vi "APC_PC_UI_Errors.vi"() -> ()   [LabVIEW 2020]
uses:
  controls/APC_ErrorCluster.ctl
  controls/APC_CylDaignosticsCluster.ctl
  <vilib>/Analysis/NI_AALBase.lvlib
panel:
  out "Clear warning request":bool
  in  "cycles for std":i32=100
  in  "Tab Control 2":enum32{"Main view", "Alternate view"}(tab)
  in  "Clear warnings":bool
  in  "Tab Control":T1(tab)=enum."CYLINDER"
  out "Round Color Box 5":u32[](array[colorbox])
  out "Round Color Box 4":u32[](array[colorbox])
  out "Round Color Box 3":u32[](array[colorbox])
  out "Round Color Box 2":u32[](array[colorbox])
  out "RASTER 5":string[](array[string])
  out "RASTER 4 : CRIO9056 : 9214-2 signals":string[](array[string])
  out "RASTER 3 : CRIO9056 : 9214-1 signals":string[](array[string])
  out "RASTER 2 : CRIO9056 : 9208 signals":string[](array[string])
  out "RASTER 1 : CRIO9056 : 9205 signals":string[](array[string])
  out "Round Color Box 1":u32[](array[colorbox])
  in  "ReloadINI9056":bool
  in  "MIN|MAX":i8[](array[numeric]) min=-1 max=1 step=1
  out "Measured value":dbl[](array[numeric])
  out "Selected raster":string[](array[string])
  in  "set9056":bool
  in  "retrieve9056":bool
  in  "Select raster":u8=1 min=1 max=5 step=1
  in  "ERROR level 2 : set IDLING":dbl[](array[numeric])
  out "Round Color Box selected":u32[](array[colorbox])
  in  "ERROR level 4: STOP and VENT":dbl[](array[numeric])
  in  "ERROR level 3 : set MOTORING":dbl[](array[numeric])
  in  "Soft WARNING level 1: self cleared":dbl[](array[numeric])
  in  "SaveINI9056":bool
  in  "Edit mode 9056":bool
  in  "Listbox":i32(listbox)
  in  "ReloadINI9049":bool
  out "s":dbl format="%#_4f"
  out "MAPO":dbl[](array[numeric])
  out "MAPO":dbl[][](graph)
  out "s":dbl format="%#_4f"
  out "s":dbl format="%#_4f"
  out "CA50":dbl[](array[numeric])
  out "CA50":dbl[][](graph)
  out "s":dbl format="%#_4f"
  out "Max p":dbl[][](graph)
  out "IMEP":dbl[][](graph)
  out "System error state":u32[][](array[colorbox])
  in  "Warning level : self cleared":dbl[](array[numeric])
  in  "Error level 2 : set MOTORING":dbl[](array[numeric])
  out "Selected raster 2":string[](array[string])=["Maximum pressure", "Misfire 1 (self reg)", "Misfire 2 (cyl to cyl)", "Misfire 3 (IMEPref)", "Cyclic variability", "MAPO", "Late combustion"]
  in  "Edit mode 9049":bool
  in  "SaveINI9049":bool
  in  "retrieve9049":bool
  in  "set9049":bool
  out "Waveform Graph":dbl[][](graph)
  out "IMEP":dbl[](array[numeric])
  out "IMEP s":dbl[](array[numeric]) format="%#.4f"
  out "Max p":dbl[](array[numeric])
  in  "EMERGENCY STOP":bool
  out "AI and system state":u32[][](array[colorbox])
  out "Cylinder pressure state":u32[][](array[colorbox])
  # "monarch APC v0.1"
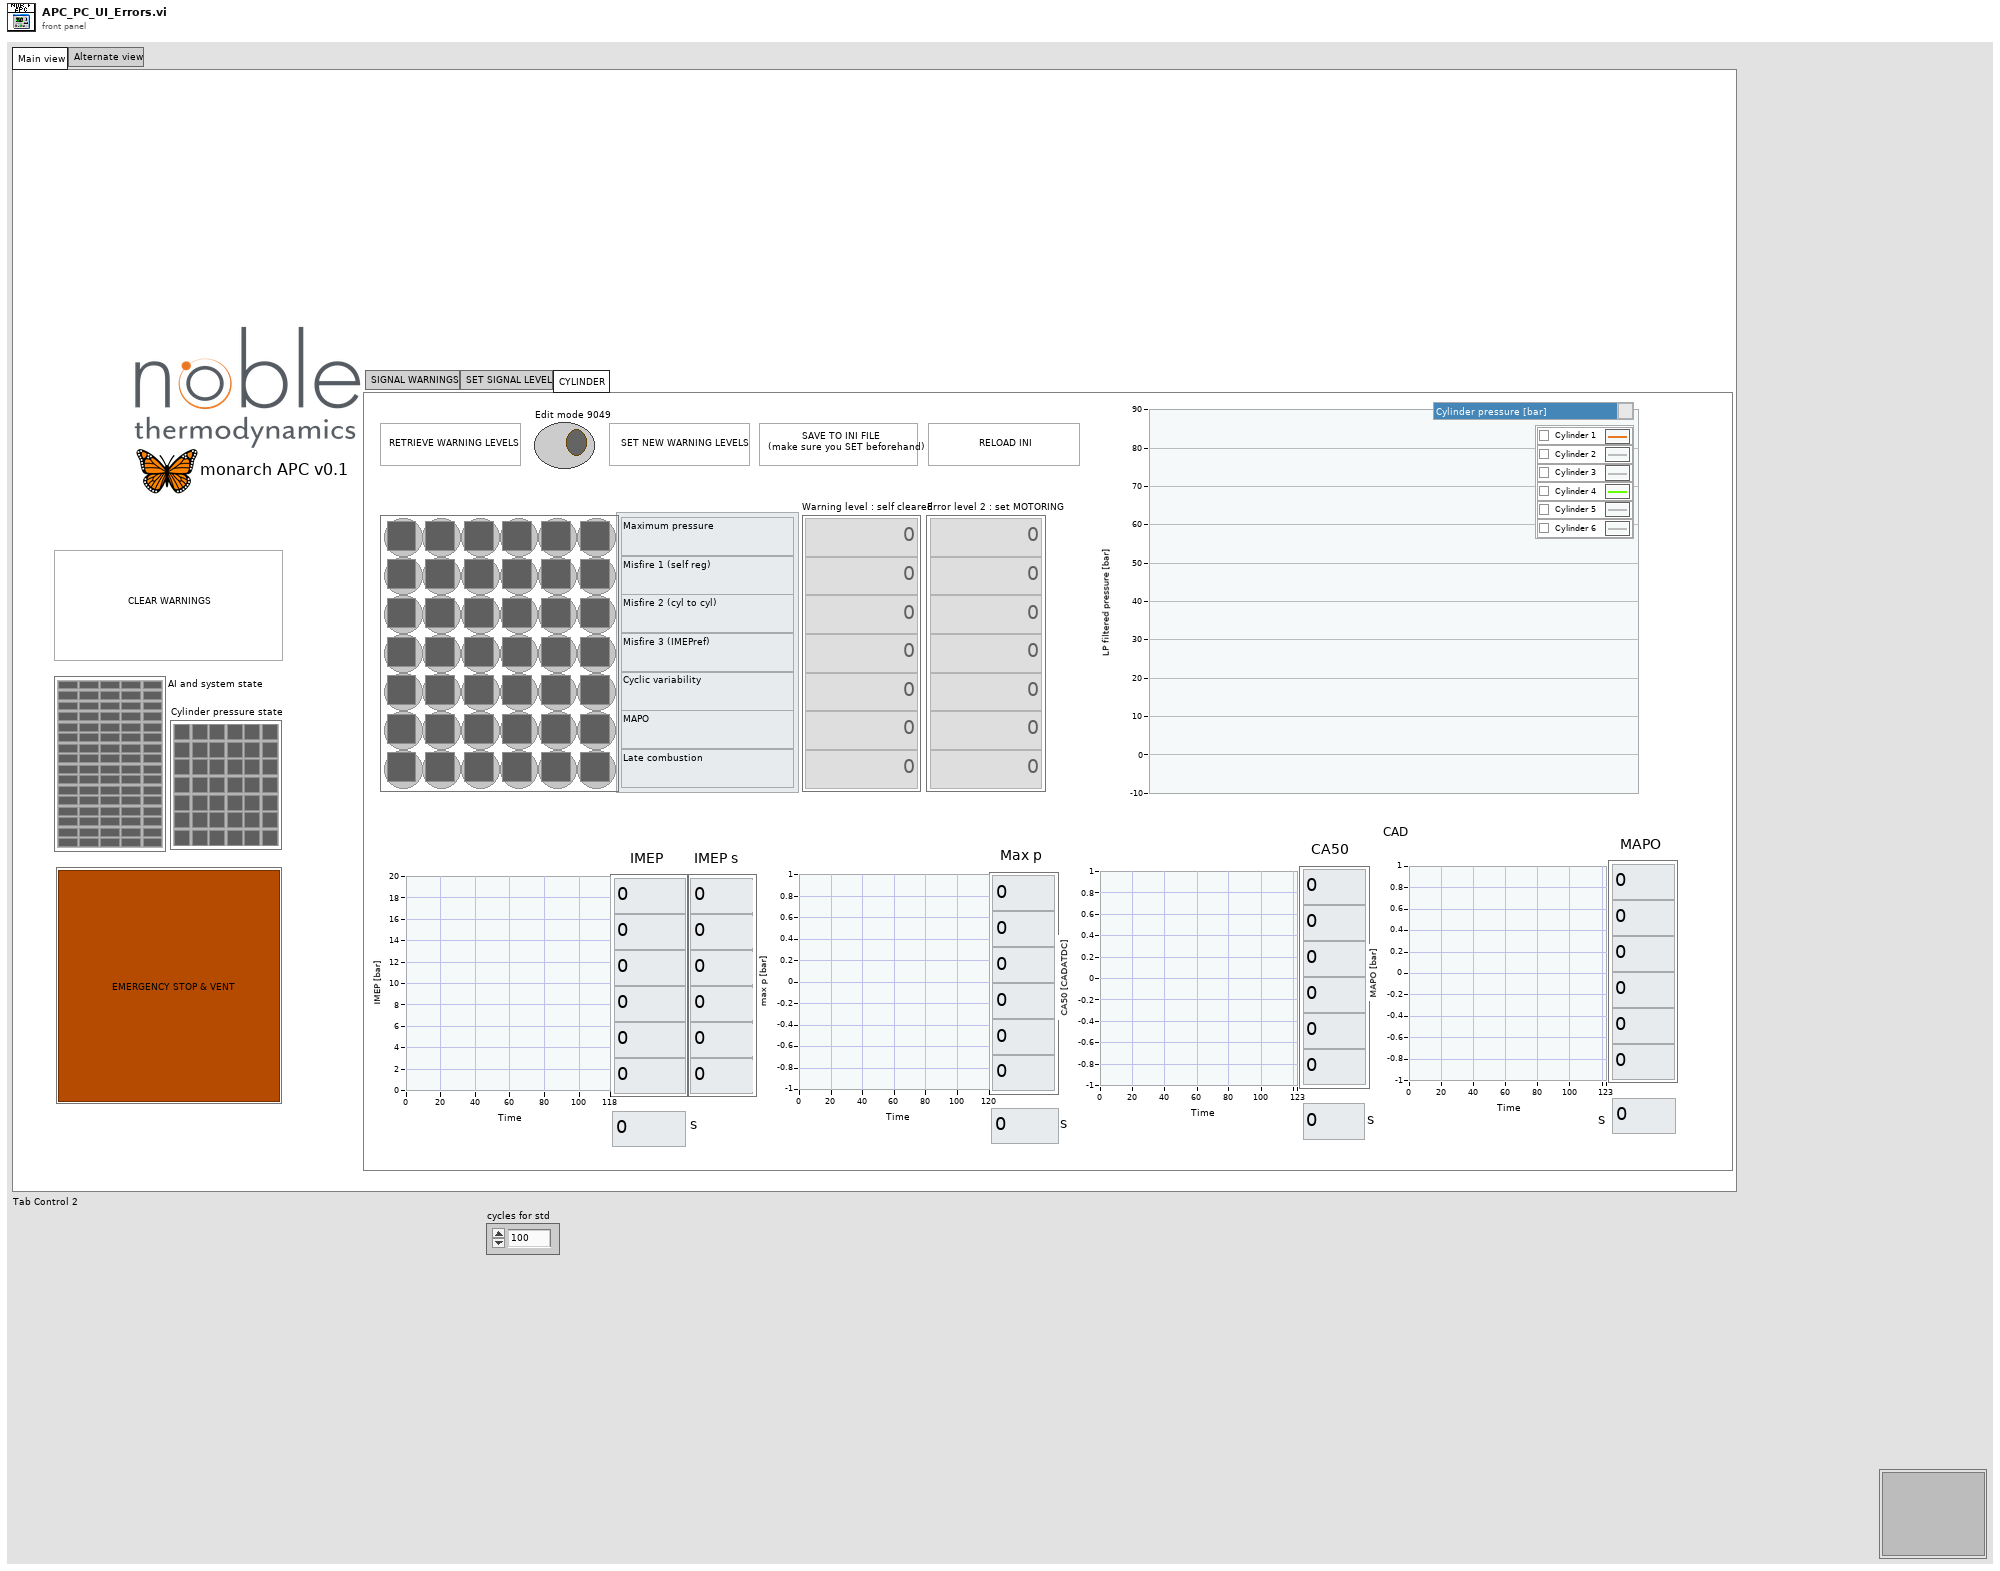
[diagram p1: front panel]
types:
  T1 = enum32{"SIGNAL WARNINGS", "SET SIGNAL LEVEL", "CYLINDER"}
  T2 = typedef "APC_ErrorCluster.ctl" = cluster{"AI and system state":u32[][], "Cylinder pressure state":u32[][], "EMERGENCY STOP":bool}
  T3 = typedef "APC_CylDaignosticsCluster.ctl" = cluster{"samples for running IMEP std":i32, "MaxDevFromExpectedIMEPError [bar]":dbl, "MaxDevFromExpectedIMEPWarning [bar]":dbl, "MaxDevFromAvgError [bar]":dbl, "MaxDevFromSelfAvgWarning [bar]":dbl, "MaxDevFromSelfAvgError [bar]":dbl, "MaxDevFromAvgWarning [bar]":dbl, "MaxIMEPstdWarning [bar]":dbl, "MaxIMEPstdError [bar]":dbl, "MAPOmaxError [bar/CAD]":dbl, "MAPOmaxWarning [bar/CAD]":dbl, "CA50maxError [CADATDC]":dbl, "CA50maxWarning [CADATDC]":dbl, "MaxPCylMaxError [bar]":dbl, "MaxPCylMaxWarning [bar]":dbl}
  T4 = typedef "APC_VisualizationCluster_v2.ctl" = cluster{"AR-FT-001":dbl, "AR-PT-001":dbl, "AR-TT-001":dbl, "AT103_CO2Conc":dbl, "AT201_CO2Conc":dbl, "C101_CompSpeed_rpm":dbl, "CO2 [%]":dbl, "EC-FC-001":dbl, "EC-TT-001":dbl, "EC-TT-002":dbl, "PC-TT-001":dbl, "PC-TT-002":dbl, "PC-TT-003":dbl, "PC-TT-004":dbl, "PC-TT-005":dbl, "PC-TT-006":dbl, "EO-PT-001":dbl, "EO-TT-001":dbl, "EO-TT-002":dbl, "FT301_Flow_kgh":dbl, "FV301_VlvPos_pc_fb":dbl, "IMEPn1":dbl, "IMEPn2":dbl, "IMEPn3":dbl, "IMEPn4":dbl, "IMEPn5":dbl, "IMEPn6":dbl, "IMEPstd1":dbl, "IMEPstd2":dbl, "IMEPstd3":dbl, "IMEPstd4":dbl, "IMEPstd5":dbl, "IMEPstd6":dbl, "NG-FC-001":dbl, "NG-FT-001":dbl, "NG-PT-001":dbl, "NG-TT-001":dbl, "NGDI-FT-001":dbl, "NGDI-PT-001":dbl, "NGDI-TT-001":dbl, "WF-OA-002-NOx":dbl, "TORQUE":dbl, "WF-OA-002-O2corr":dbl, "O2-FC-001":dbl, "O2-PT-001":dbl, "O2-TT-001":dbl, "PT103_Pressure_kPa":dbl, "PT104_Pressure_kPa":dbl, "PT106_Pressure_kPa":dbl, "PT300_Pressure_kPa":dbl, "PV103_VlvPos_pc_fb":dbl, "PV300_VlvPos_pc_fb":dbl, "MaxPcyl1":dbl, "MaxPcyl2":dbl, "MaxPcyl3":dbl, "MaxPcyl4":dbl, "MaxPcyl5":dbl, "MaxPcyl6":dbl, "SW-FC-004":dbl, "SW-FC-009":dbl, "SW-FT-001":dbl, "SW-FT-002":dbl, "SW-FT-003":dbl, "SW-FT-004":dbl, "SW-TT-001":dbl, "SW-TT-002":dbl, "SW-TT-003":dbl, "SW-TT-004":dbl, "SW-TT-005":dbl, "SW-TT-006":dbl, "SW-TT-007":dbl, "SW-TT-008":dbl, "WF-OA-001":dbl, "WF-OA-002":dbl, "WF-PT-001":dbl, "WF-PT-004":dbl, "WF-PT-005avg":dbl, "WF-PT-014":dbl, "WF-PT-015":dbl, "WF-PT-016":dbl, "WF-TT-001":dbl, "WF-TT-002":dbl, "WF-TT-003":dbl, "WF-TT-004":dbl, "WF-TT-007":dbl, "EngineSpeed_rpm":dbl, "SystemState":dbl, "CylPresWarnings":dbl, "CylPresErrors":dbl, "MAPO1":dbl, "MAPO2":dbl, "MAPO3":dbl, "MAPO4":dbl, "MAPO5":dbl, "MAPO6":dbl, "CA50_1":dbl, "CA50_2":dbl, "CA50_3":dbl, "CA50_4":dbl, "CA50_5":dbl, "CA50_6":dbl, "SparkTiming":dbl, "SW-TT-009":dbl, "NG-FV-001":dbl, "O2-PV-004":dbl, "AR-PV-004":dbl, "WF-FC-001":dbl, "WF-FC-002":dbl, "WF-FC-003":dbl, "WF-PT-012avg":dbl}
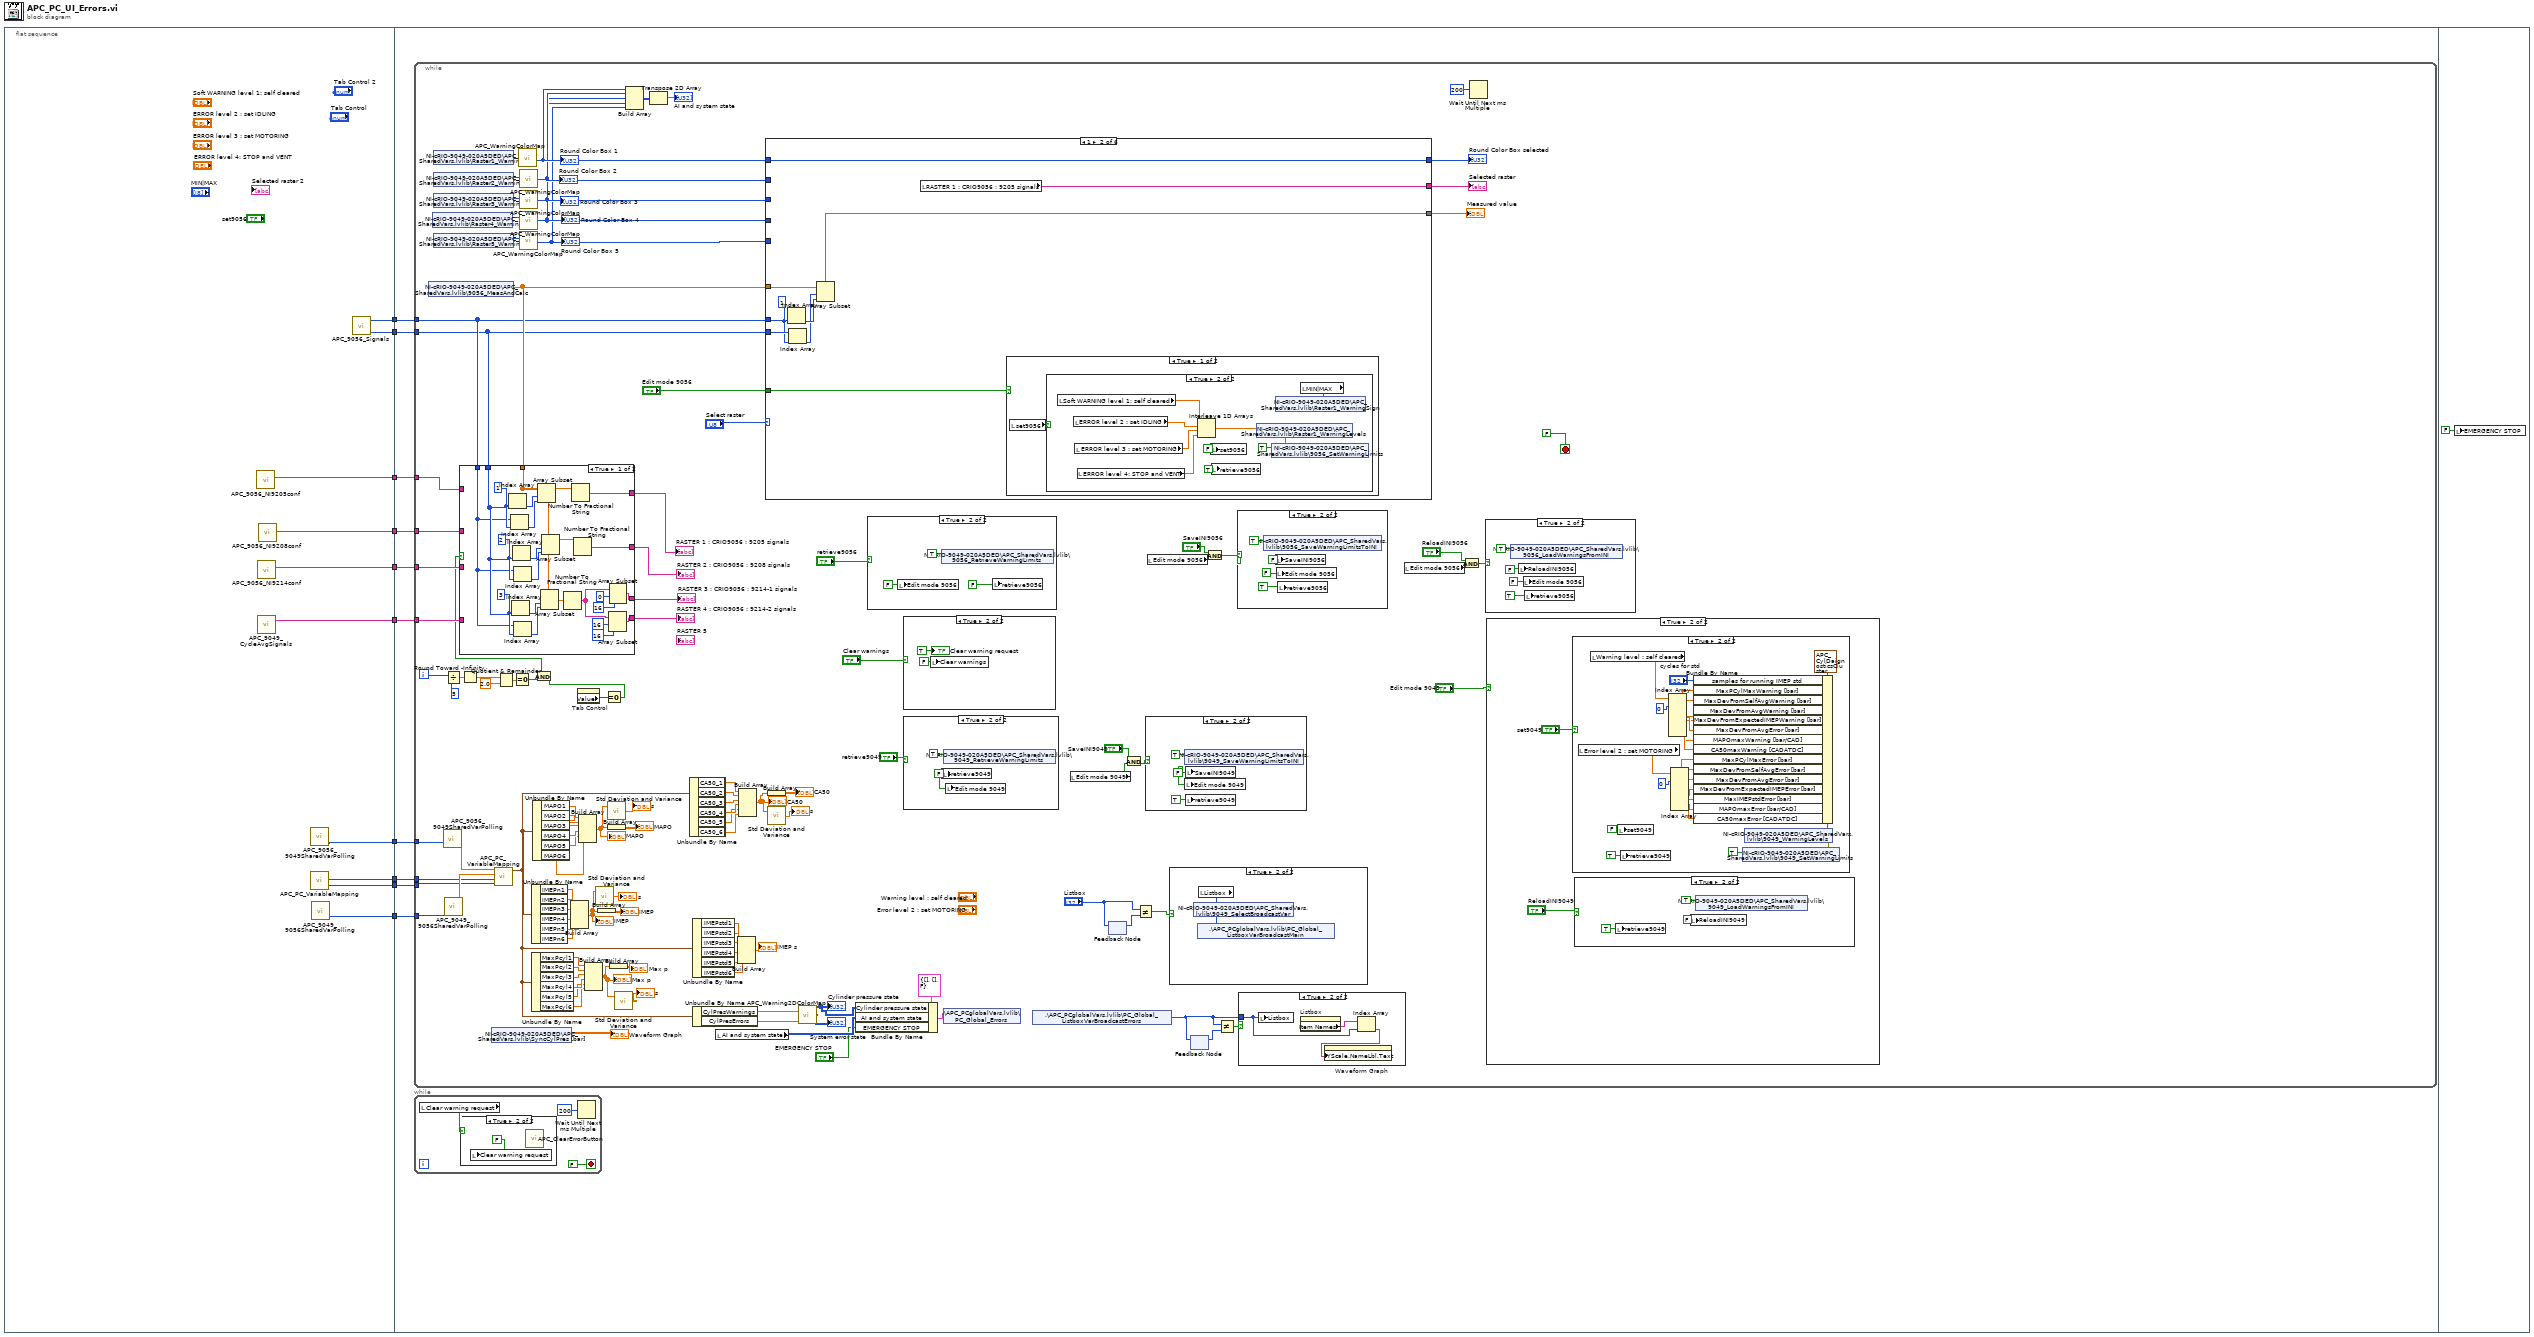
[diagram p0: block diagram]
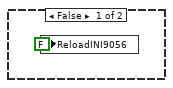
[diagram p5: hidden frame]
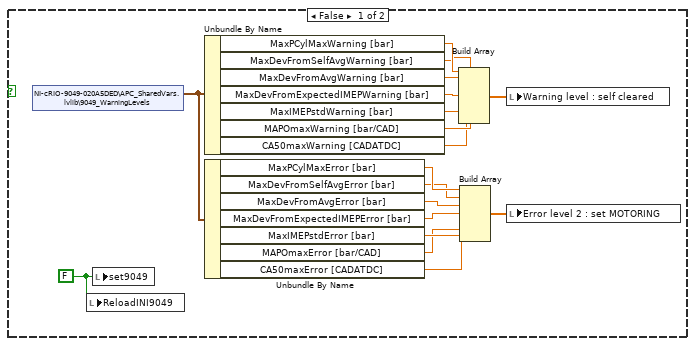
[diagram p6: hidden frame]
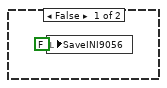
[diagram p13: hidden frame]
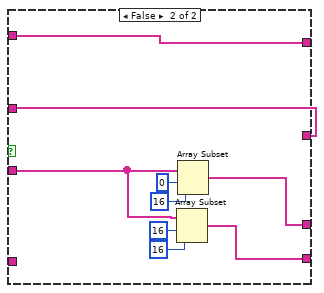
[diagram p14: hidden frame]
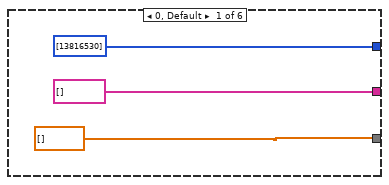
[diagram p15: hidden frame]
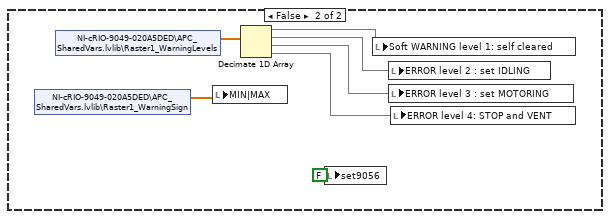
[diagram p17: hidden frame]
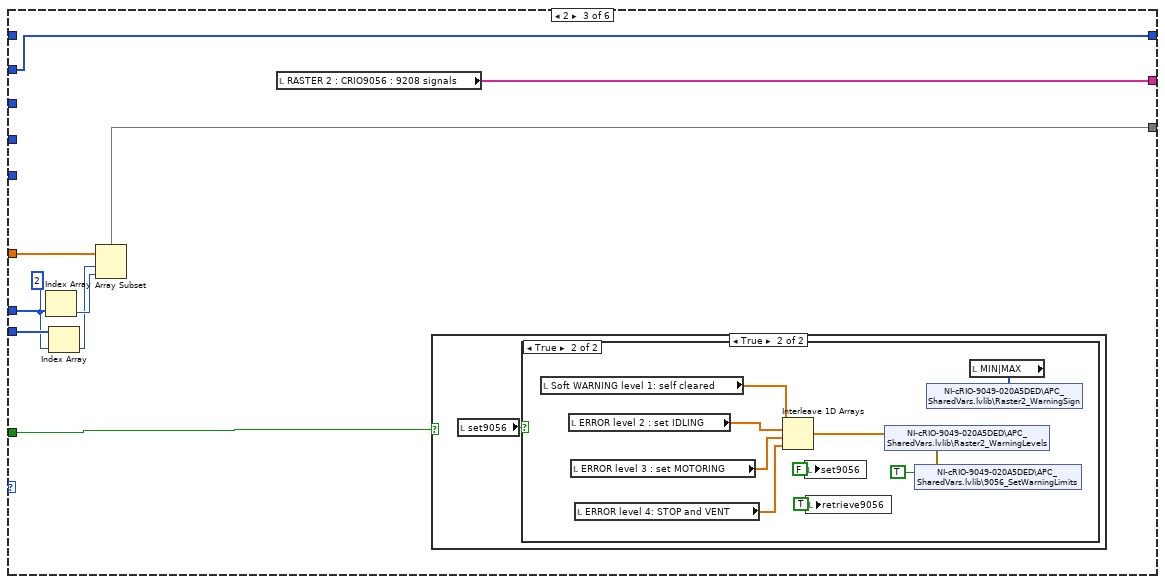
[diagram p18: hidden frame]
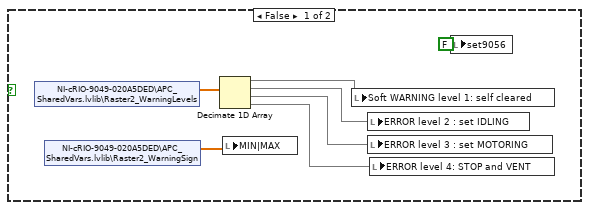
[diagram p19: hidden frame]
diagram:
  n1 = flat-sequence {
    tunnel: [w20] -> w10
    tunnel: [w19] -> w9
    tunnel: [w18] -> w8
    tunnel: [w17] -> w7
    tunnel: [w16] -> w6
    tunnel: [w15] -> w5
    tunnel: [w14] -> w4
    tunnel: [w13] -> w3
    tunnel: [w12] -> w2
    tunnel: [w11] -> w1
    tunnel: w10 -> [w30]
    tunnel: w9 -> [w29]
    tunnel: w8 -> [w28]
    tunnel: w7 -> [w27]
    tunnel: w6 -> [w26]
    tunnel: w5 -> [w25]
    tunnel: w4 -> [w24]
    tunnel: w3 -> [w23]
    tunnel: w2 -> [w22]
    tunnel: w1 -> [w21]
    frame #0 {
      n2 = call "APC_9056_NI9205conf.vi"() -> ("channels name out"=w18:string[])  [unwired: 5 out]
      n3 = call "APC_9056_NI9214conf.vi"() -> ("channels name out"=w16:string[])  [unwired: 5 in]
      n4 = call "APC_9049_CycleAvgSignals.vi"() -> ("CRIo9049_CycleAvgSignals"=w15:string[])  [unwired: 3 in]
      n5 = call "APC_9056_NI9208conf.vi"() -> ("channels name out"=w17:string[])  [unwired: 5 out]
      n6 = call "APC_9056_9049SharedVarPolling.vi"() -> ("Number of signals (out)"=w14:i32)  [unwired: 1 in, 1 out]
      n7 = call "APC_PC_VariableMapping.vi"() -> ("Index 9056"=w11:i32[], "Index 9049"=w12:i32[])  [unwired: 4 in, 1 out]
      n8 = call "APC_9049_9056SharedVarPolling.vi"() -> ("Number of signals (out)"=w13:i32)  [unwired: 1 in, 3 out]
      n9 = call "APC_9056_Signals.vi"() -> ("Starting Index"=w19:i32[], "signals per group"=w20:i32[])  [unwired: 3 in, 1 out]
    }
    frame #1 {
      n10 = while {
        tunnel: w30 -> [w124]
        tunnel: w29 -> [w123]
        tunnel: w28 -> [w136]
        tunnel: w27 -> [w135]
        tunnel: w26 -> [w134]
        tunnel: w25 -> [w133]
        tunnel: w24 -> [w114]
        tunnel: w23 -> [w113]
        tunnel: w22 -> [w112]
        tunnel: w21 -> [w111]
        i -> [w142]
        stop <- FALSE stop-if-true
        n11 = shared-variable "NI-cRIO-9049-020A5DED\\APC_SharedVars.lvlib\\9056_MeasAndCalc"() -> (w128:dbl[])  [unwired: 1 in, 1 out]
        n12 = shared-variable "NI-cRIO-9049-020A5DED\\APC_SharedVars.lvlib\\Raster4_Warnings"() -> (w146:u8[])  [unwired: 1 in, 1 out]
        n13 = shared-variable "NI-cRIO-9049-020A5DED\\APC_SharedVars.lvlib\\Raster1_Warnings"() -> (w149:u8[])  [unwired: 1 in, 1 out]
        n14 = shared-variable "NI-cRIO-9049-020A5DED\\APC_SharedVars.lvlib\\Raster2_Warnings"() -> (w148:u8[])  [unwired: 1 in, 1 out]
        n15 = shared-variable "NI-cRIO-9049-020A5DED\\APC_SharedVars.lvlib\\Raster3_Warnings"() -> (w147:u8[])  [unwired: 1 in, 1 out]
        n16 = shared-variable "NI-cRIO-9049-020A5DED\\APC_SharedVars.lvlib\\Raster5_Warnings"() -> (w145:u8[])  [unwired: 1 in, 1 out]
        n17 = call "APC_9056_9049SharedVarPolling.vi"("Number of signals"=w114) -> ("9049_CycleAveragedVariables"=w116:dbl[])  [unwired: 1 out]
        n18 = call "APC_9049_9056SharedVarPolling.vi"("Number of signals"=w113) -> ("9056 IO"=w115:dbl[])  [unwired: 3 out]
        n19 = Divide(x=w142, y=5) -> (x/y=w140:dbl)
        n20 = Round Toward -Infinity(1:w140) -> (0:w139:dbl)
        n21 = shared-variable "NI-cRIO-9049-020A5DED\\APC_SharedVars.lvlib\\SyncCylPres [bar]"() -> (→"Waveform Graph":dbl[][])  [unwired: 1 in, 1 out]
        n22 = call "APC_PC_VariableMapping.vi"("Index of array for 9056"=w111, "Index of array for 9049"=w112, "9056 IO"=w115, "9049_CycleAveragedVariables"=w116) -> ("Output cluster"=w85:T4)  [unwired: 2 out]
        n23 = Quotient & Remainder(x=w139, y=2.0) -> (x-y*floor(x/y)=w137:dbl)  [unwired: 1 out]
        n24 = Equal To 0?(x=w137) -> (x = 0?=w127:bool)
        n25 = call "APC_WarningColorMap.vi"("Array"=w149) -> ("Round Color Box"=w67:u32[])
        "Round Color Box 1" <- w67
        n26 = call "APC_WarningColorMap.vi"("Array"=w148) -> ("Round Color Box"=w66:u32[])
        "Round Color Box 2" <- w66
        n27 = call "APC_WarningColorMap.vi"("Array"=w147) -> ("Round Color Box"=w65:u32[])
        "Round Color Box 3" <- w65
        n28 = call "APC_WarningColorMap.vi"("Array"=w146) -> ("Round Color Box"=w64:u32[])
        "Round Color Box 4" <- w64
        n29 = call "APC_WarningColorMap.vi"("Array"=w145) -> ("Round Color Box"=w63:u32[])
        "Round Color Box 5" <- w63
        n30 = Unbundle By Name(w85) -> ("IMEPn1"=w109:dbl, "IMEPn2"=w104:dbl, "IMEPn3"=w105:dbl, "IMEPn4"=w106:dbl, "IMEPn5"=w107:dbl, "IMEPn6"=w108:dbl)
        n31 = Unbundle By Name(w85) -> ("MaxPcyl1"=w96:dbl, "MaxPcyl2"=w95:dbl, "MaxPcyl3"=w94:dbl, "MaxPcyl4"=w93:dbl, "MaxPcyl5"=w92:dbl, "MaxPcyl6"=w91:dbl)
        n32 = Unbundle By Name(w85) -> ("MAPO1"=w83:dbl, "MAPO2"=w82:dbl, "MAPO3"=w81:dbl, "MAPO4"=w80:dbl, "MAPO5"=w79:dbl, "MAPO6"=w78:dbl)
        n33 = Build Array(w109, w104, w105, w106, w107, w108) -> (w60:dbl[])
        "IMEP" <- w60
        n34 = property on="Tab Control" class="TabCtl (strict)"() -> ("Value"=w121:T1)  [unwired: 2 in, 2 out]
        n35 = Build Array(w83, w82, w81, w80, w79, w78) -> (w47:dbl[])
        "MAPO" <- w47
        n36 = Build Array(w96, w95, w94, w93, w92, w91) -> (w43:dbl[])
        "Max p" <- w43
        n37 = call <vilib>:"Std Deviation and Variance.vi"("X"=w60) -> ("standard deviation"=→"s":dbl)  [unwired: 1 in, 2 out]
        n38 = Build Array(w60) -> (→"IMEP":dbl[][])
        n39 = Equal To 0?(x=w121) -> (x = 0?=w125:bool)
        n40 = And(x=w125, y=w127) -> (x .and. y?=w126:bool)
        n41 = case shown="True" w126 {
          tunnel: [w234 w256] -> w132
          tunnel: w136 -> [_ w256]
          tunnel: [w232 w255] -> w131
          tunnel: w135 -> [_ w255]
          tunnel: [w224 w254] -> w130
          tunnel: w134 -> [_ w249]
          tunnel: [w225 w248] -> w129
          tunnel: w133 -> [_ _]
          tunnel: w128 -> [w236 _]
          tunnel: w123 -> [w238 _]
          tunnel: w124 -> [w237 _]
          frame True {
            w239 = 3 ("index")
            w242 = 2 ("index")
            w245 = 1 ("index")
            n42 = Index Array(array=w238, index=w245) -> (element=w247:i32)
            n43 = Index Array(array=w237, index=w245) -> (element=w246:i32)
            n44 = Index Array(array=w238, index=w239) -> (element=w241:i32)
            n45 = Index Array(array=w238, index=w242) -> (element=w244:i32)
            n46 = Index Array(array=w237, index=w239) -> (element=w240:i32)
            n47 = Index Array(array=w237, index=w242) -> (element=w243:i32)
            n48 = Array Subset(array=w236, index=w247, length=w246) -> (w235:dbl[])
            n49 = Array Subset(array=w236, index=w241, length=w240) -> (w231:dbl[])
            n50 = Array Subset(array=w236, index=w244, length=w243) -> (w233:dbl[])
            n51 = Number To Fractional String(number=w231) -> (F-format string=w226:string[])  [unwired: 3 in]
            n52 = Number To Fractional String(number=w235) -> (F-format string=w234:string[])  [unwired: 3 in]
            n53 = Number To Fractional String(number=w233) -> (F-format string=w232:string[])  [unwired: 3 in]
            n54 = Array Subset(array=w226, index=16, length=16) -> (w225:string[])
            n55 = Array Subset(array=w226, index=0, length=16) -> (w224:string[])
          }
          frame False {
            n56 = Array Subset(array=w249, index=16, length=16) -> (w248:string[])
            n57 = Array Subset(array=w249, index=0, length=16) -> (w254:string[])
          }
        }
        "RASTER 1 : CRIO9056 : 9205 signals" <- w132
        "RASTER 2 : CRIO9056 : 9208 signals" <- w131
        "RASTER 3 : CRIO9056 : 9214-1 signals" <- w130
        "RASTER 4 : CRIO9056 : 9214-2 signals" <- w129
        n58 = Build Array(w47) -> (→"MAPO":dbl[][])
        n59 = call <vilib>:"Std Deviation and Variance.vi"("X"=w47) -> ("standard deviation"=→"s":dbl)  [unwired: 1 in, 2 out]
        n60 = Build Array(w43) -> (→"Max p":dbl[][])
        n61 = call <vilib>:"Std Deviation and Variance.vi"("X"=w43) -> ("standard deviation"=→"s":dbl)  [unwired: 1 in, 2 out]
        n62 = Build Array(w67, w66, w65, w64, w63) -> (w62:u32[][])
        n63 = Transpose 2D Array(2D array=w62) -> (transposed array=→"AI and system state":u32[][])
        n64 = Unbundle By Name(w85) -> ("CA50_1"=w84:dbl, "CA50_2"=w90:dbl, "CA50_3"=w89:dbl, "CA50_4"=w88:dbl, "CA50_5"=w87:dbl, "CA50_6"=w86:dbl)
        n65 = Unbundle By Name(w85) -> ("IMEPstd1"=w103:dbl, "IMEPstd2"=w102:dbl, "IMEPstd3"=w101:dbl, "IMEPstd4"=w100:dbl, "IMEPstd5"=w99:dbl, "IMEPstd6"=w98:dbl)
        n66 = Unbundle By Name(w85) -> ("CylPresWarnings"=w77:dbl, "CylPresErrors"=w76:dbl)
        n67 = local read "AI and system state"() -> (w39:u32[][])
        n68 = Build Array(w103, w102, w101, w100, w99, w98) -> (→"IMEP s":dbl[])
        n69 = Build Array(w84, w90, w89, w88, w87, w86) -> (w46:dbl[])
        "CA50" <- w46
        n70 = case shown="1" "Select raster" {
          tunnel: w67 -> [_ w269 _ _ _ _]
          tunnel: w66 -> [_ _ w289 _ _ _]
          tunnel: w65 -> [_ _ _ w318 _ _]
          tunnel: w64 -> [_ _ _ _ w349 _]
          tunnel: w63 -> [_ _ _ _ _ w375]
          tunnel: [u32[] [13816530] ("Round Color Box") w269 w289 w318 w349 w375] -> w150
          tunnel: [string[] [] ("RASTER 5") w268 w297 w325 w355 w383] -> w144
          tunnel: [dbl[] [] ("Measured value") w263 w292 w320 w350 w378] -> w143
          tunnel: w128 -> [_ w267 w296 w324 w354 w382]
          tunnel: w124 -> [_ w266 w295 w323 w353 w381]
          tunnel: w123 -> [_ w265 w294 w322 w352 w380]
          tunnel: "Edit mode 9056" -> [_ w260 w288 w317 w348 w374]
          frame 0, Default {
          }
          frame 1 {
            w264 = 1 ("index")
            n71 = Index Array(array=w266, index=w264) -> (element=w262:i32)
            n72 = Index Array(array=w265, index=w264) -> (element=w261:i32)
            n73 = Array Subset(array=w267, index=w261, length=w262) -> (w263:dbl[])
            n74 = local read "RASTER 1 : CRIO9056 : 9205 signals"() -> (w268:string[])
            n75 = case shown="True" w260 {
              frame True {
                n76 = local read "set9056"() -> (w270:bool)
                n77 = case shown="True" w270 {
                  frame False {
                  }
                  frame True {
                    n78 = local read "Soft WARNING level 1: self cleared"() -> (w276:dbl[])
                    n79 = local read "ERROR level 2 : set IDLING"() -> (w275:dbl[])
                    n80 = local read "ERROR level 3 : set MOTORING"() -> (w274:dbl[])
                    n81 = local read "ERROR level 4: STOP and VENT"() -> (w273:dbl[])
                    n82 = Interleave 1D Arrays(w276, w275, w274, w273) -> (w272:dbl[])
                    n83 = local write "set9056"(FALSE ("set")) -> ()
                    n84 = local write "retrieve9056"(TRUE ("retrieve")) -> ()
                    n85 = shared-variable "NI-cRIO-9049-020A5DED\\APC_SharedVars.lvlib\\Raster1_WarningLevels"(w272) -> (error out=w277:errorcluster)  [unwired: 1 in]
                    n86 = shared-variable "NI-cRIO-9049-020A5DED\\APC_SharedVars.lvlib\\9056_SetWarningLimits"(TRUE ("SetWarningLimits"), error in=w277) -> ()  [unwired: 1 out]
                    n87 = local read "MIN|MAX"() -> (w271:i8[])
                    n88 = shared-variable "NI-cRIO-9049-020A5DED\\APC_SharedVars.lvlib\\Raster1_WarningSign"(w271) -> ()  [unwired: 1 in, 1 out]
                  }
                }
              }
              frame False {
                n89 = shared-variable "NI-cRIO-9049-020A5DED\\APC_SharedVars.lvlib\\Raster1_WarningSign"() -> (w282:dbl[])  [unwired: 1 in, 1 out]
                n90 = shared-variable "NI-cRIO-9049-020A5DED\\APC_SharedVars.lvlib\\Raster1_WarningLevels"() -> (w287:dbl[])  [unwired: 1 in, 1 out]
                n91 = local write "MIN|MAX"(w282) -> ()
                n92 = Decimate 1D Array(w287) -> (w286:dbl[], w285:dbl[], w284:dbl[], w283:dbl[])
                n93 = local write "set9056"(FALSE ("set")) -> ()
                n94 = local write "Soft WARNING level 1: self cleared"(w286) -> ()
                n95 = local write "ERROR level 2 : set IDLING"(w285) -> ()
                n96 = local write "ERROR level 3 : set MOTORING"(w284) -> ()
                n97 = local write "ERROR level 4: STOP and VENT"(w283) -> ()
              }
            }
          }
          frame 2 {
            w293 = 2 ("index")
            n98 = Index Array(array=w295, index=w293) -> (element=w291:i32)
            n99 = Index Array(array=w294, index=w293) -> (element=w290:i32)
            n100 = Array Subset(array=w296, index=w290, length=w291) -> (w292:dbl[])
            n101 = local read "RASTER 2 : CRIO9056 : 9208 signals"() -> (w297:string[])
            n102 = case shown="True" w288 {
              frame False {
                n103 = shared-variable "NI-cRIO-9049-020A5DED\\APC_SharedVars.lvlib\\Raster2_WarningLevels"() -> (w300:dbl[])  [unwired: 1 in, 1 out]
                n104 = shared-variable "NI-cRIO-9049-020A5DED\\APC_SharedVars.lvlib\\Raster2_WarningSign"() -> (w299:dbl[])  [unwired: 1 in, 1 out]
                n105 = Decimate 1D Array(w300) -> (w301:dbl[], w302:dbl[], w303:dbl[], w304:dbl[])
                n106 = local write "MIN|MAX"(w299) -> ()
                n107 = local write "Soft WARNING level 1: self cleared"(w301) -> ()
                n108 = local write "ERROR level 2 : set IDLING"(w302) -> ()
                n109 = local write "ERROR level 3 : set MOTORING"(w303) -> ()
                n110 = local write "ERROR level 4: STOP and VENT"(w304) -> ()
                n111 = local write "set9056"(FALSE ("set")) -> ()
              }
              frame True {
                n112 = local read "set9056"() -> (w305:bool)
                n113 = case shown="True" w305 {
                  frame False {
                  }
                  frame True {
                    n114 = local read "Soft WARNING level 1: self cleared"() -> (w311:dbl[])
                    n115 = local read "ERROR level 2 : set IDLING"() -> (w310:dbl[])
                    n116 = local read "ERROR level 3 : set MOTORING"() -> (w309:dbl[])
                    n117 = local read "ERROR level 4: STOP and VENT"() -> (w308:dbl[])
                    n118 = Interleave 1D Arrays(w311, w310, w309, w308) -> (w307:dbl[])
                    n119 = local write "set9056"(FALSE ("set")) -> ()
                    n120 = local write "retrieve9056"(TRUE ("retrieve")) -> ()
                    n121 = shared-variable "NI-cRIO-9049-020A5DED\\APC_SharedVars.lvlib\\Raster2_WarningLevels"(w307) -> (error out=w312:errorcluster)  [unwired: 1 in]
                    n122 = shared-variable "NI-cRIO-9049-020A5DED\\APC_SharedVars.lvlib\\9056_SetWarningLimits"(TRUE ("SetWarningLimits"), error in=w312) -> ()  [unwired: 1 out]
                    n123 = local read "MIN|MAX"() -> (w306:i8[])
                    n124 = shared-variable "NI-cRIO-9049-020A5DED\\APC_SharedVars.lvlib\\Raster2_WarningSign"(w306) -> ()  [unwired: 1 in, 1 out]
                  }
                }
              }
            }
          }
          frame 3 {
            w321 = 3 ("index")
            n125 = Index Array(array=w323, index=w321) -> ()  [unwired: 1 out]
            n126 = Index Array(array=w322, index=w321) -> (element=w319:i32)
            n127 = Array Subset(array=w324, index=w319, length=16) -> (w320:dbl[])
            n128 = local read "RASTER 3 : CRIO9056 : 9214-1 signals"() -> (w325:string[])
            n129 = case shown="True" w317 {
              frame True {
                n130 = local read "set9056"() -> (w326:bool)
                n131 = case shown="True" w326 {
                  frame False {
                  }
                  frame True {
                    n132 = local read "Soft WARNING level 1: self cleared"() -> (w332:dbl[])
                    n133 = local read "ERROR level 2 : set IDLING"() -> (w331:dbl[])
                    n134 = local read "ERROR level 3 : set MOTORING"() -> (w330:dbl[])
                    n135 = local read "ERROR level 4: STOP and VENT"() -> (w329:dbl[])
                    n136 = Interleave 1D Arrays(w332, w331, w330, w329) -> (w328:dbl[])
                    n137 = local write "set9056"(FALSE ("set")) -> ()
                    n138 = local write "retrieve9056"(TRUE ("retrieve")) -> ()
                    n139 = shared-variable "NI-cRIO-9049-020A5DED\\APC_SharedVars.lvlib\\Raster3_WarningLevels"(w328) -> (error out=w333:errorcluster)  [unwired: 1 in]
                    n140 = shared-variable "NI-cRIO-9049-020A5DED\\APC_SharedVars.lvlib\\9056_SetWarningLimits"(TRUE ("SetWarningLimits"), error in=w333) -> ()  [unwired: 1 out]
                    n141 = local read "MIN|MAX"() -> (w327:i8[])
                    n142 = shared-variable "NI-cRIO-9049-020A5DED\\APC_SharedVars.lvlib\\Raster3_WarningSign"(w327) -> ()  [unwired: 1 in, 1 out]
                  }
                }
              }
              frame False {
                n143 = shared-variable "NI-cRIO-9049-020A5DED\\APC_SharedVars.lvlib\\Raster3_WarningSign"() -> (w338:dbl[])  [unwired: 1 in, 1 out]
                n144 = shared-variable "NI-cRIO-9049-020A5DED\\APC_SharedVars.lvlib\\Raster3_WarningLevels"() -> (w343:dbl[])  [unwired: 1 in, 1 out]
                n145 = local write "MIN|MAX"(w338) -> ()
                n146 = Decimate 1D Array(w343) -> (w342:dbl[], w341:dbl[], w340:dbl[], w339:dbl[])
                n147 = local write "Soft WARNING level 1: self cleared"(w342) -> ()
                n148 = local write "ERROR level 2 : set IDLING"(w341) -> ()
                n149 = local write "ERROR level 3 : set MOTORING"(w340) -> ()
                n150 = local write "ERROR level 4: STOP and VENT"(w339) -> ()
                n151 = local write "set9056"(FALSE ("set")) -> ()
              }
            }
          }
          frame 4 {
            w351 = 3 ("index")
            n152 = Index Array(array=w353, index=w351) -> ()  [unwired: 1 out]
            n153 = Index Array(array=w352, index=w351) -> (element=w345:i32)
            n154 = Add(x=w345, y=16) -> (x+y=w346:i32)
            n155 = Array Subset(array=w354, index=w346, length=16) -> (w350:dbl[])
            n156 = local read "RASTER 4 : CRIO9056 : 9214-2 signals"() -> (w355:string[])
            n157 = case shown="False" w348 {
              frame True {
                n158 = local read "set9056"() -> (w356:bool)
                n159 = case shown="True" w356 {
                  frame False {
                  }
                  frame True {
                    n160 = local read "Soft WARNING level 1: self cleared"() -> (w362:dbl[])
                    n161 = local read "ERROR level 2 : set IDLING"() -> (w361:dbl[])
                    n162 = local read "ERROR level 3 : set MOTORING"() -> (w360:dbl[])
                    n163 = local read "ERROR level 4: STOP and VENT"() -> (w359:dbl[])
                    n164 = Interleave 1D Arrays(w362, w361, w360, w359) -> (w358:dbl[])
                    n165 = local write "set9056"(FALSE ("set")) -> ()
                    n166 = local write "retrieve9056"(TRUE ("retrieve")) -> ()
                    n167 = shared-variable "NI-cRIO-9049-020A5DED\\APC_SharedVars.lvlib\\Raster4_WarningLevels"(w358) -> (error out=w363:errorcluster)  [unwired: 1 in]
                    n168 = local read "MIN|MAX"() -> (w357:i8[])
                    n169 = shared-variable "NI-cRIO-9049-020A5DED\\APC_SharedVars.lvlib\\Raster4_WarningSign"(w357) -> ()  [unwired: 1 in, 1 out]
                    n170 = shared-variable "NI-cRIO-9049-020A5DED\\APC_SharedVars.lvlib\\9056_SetWarningLimits"(TRUE ("SetWarningLimits"), error in=w363) -> ()  [unwired: 1 out]
                  }
                }
              }
              frame False {
                n171 = shared-variable "NI-cRIO-9049-020A5DED\\APC_SharedVars.lvlib\\Raster4_WarningSign"() -> (w368:dbl[])  [unwired: 1 in, 1 out]
                n172 = shared-variable "NI-cRIO-9049-020A5DED\\APC_SharedVars.lvlib\\Raster4_WarningLevels"() -> (w373:dbl[])  [unwired: 1 in, 1 out]
                n173 = local write "MIN|MAX"(w368) -> ()
                n174 = Decimate 1D Array(w373) -> (w372:dbl[], w371:dbl[], w370:dbl[], w369:dbl[])
                n175 = local write "Soft WARNING level 1: self cleared"(w372) -> ()
                n176 = local write "ERROR level 2 : set IDLING"(w371) -> ()
                n177 = local write "ERROR level 3 : set MOTORING"(w370) -> ()
                n178 = local write "ERROR level 4: STOP and VENT"(w369) -> ()
                n179 = local write "set9056"(FALSE ("set")) -> ()
              }
            }
          }
          frame 5 {
            w379 = 5 ("index")
            n180 = Index Array(array=w381, index=w379) -> (element=w377:i32)
            n181 = Index Array(array=w380, index=w379) -> (element=w376:i32)
            n182 = Array Subset(array=w382, index=w376, length=w377) -> (w378:dbl[])
            n183 = local read "RASTER 5"() -> (w383:string[])
            n184 = case shown="False" w374 {
              frame True {
                n185 = local read "set9056"() -> (w384:bool)
                n186 = case shown="True" w384 {
                  frame False {
                  }
                  frame True {
                    n187 = local read "Soft WARNING level 1: self cleared"() -> (w390:dbl[])
                    n188 = local read "ERROR level 2 : set IDLING"() -> (w389:dbl[])
                    n189 = local read "ERROR level 3 : set MOTORING"() -> (w388:dbl[])
                    n190 = local read "ERROR level 4: STOP and VENT"() -> (w387:dbl[])
                    n191 = Interleave 1D Arrays(w390, w389, w388, w387) -> (w386:dbl[])
                    n192 = local write "set9056"(FALSE ("set")) -> ()
                    n193 = local write "retrieve9056"(TRUE ("retrieve")) -> ()
                    n194 = shared-variable "NI-cRIO-9049-020A5DED\\APC_SharedVars.lvlib\\Raster5_WarningLevels"(w386) -> (error out=w391:errorcluster)  [unwired: 1 in]
                    n195 = local read "MIN|MAX"() -> (w385:i8[])
                    n196 = shared-variable "NI-cRIO-9049-020A5DED\\APC_SharedVars.lvlib\\Raster5_WarningSign"(w385) -> ()  [unwired: 1 in, 1 out]
                    n197 = shared-variable "NI-cRIO-9049-020A5DED\\APC_SharedVars.lvlib\\9056_SetWarningLimits"(TRUE ("SetWarningLimits"), error in=w391) -> ()  [unwired: 1 out]
                  }
                }
              }
              frame False {
                n198 = shared-variable "NI-cRIO-9049-020A5DED\\APC_SharedVars.lvlib\\Raster5_WarningSign"() -> (w396:dbl[])  [unwired: 1 in, 1 out]
                n199 = shared-variable "NI-cRIO-9049-020A5DED\\APC_SharedVars.lvlib\\Raster5_WarningLevels"() -> (w397:dbl[])  [unwired: 1 in, 1 out]
                n200 = local write "MIN|MAX"(w396) -> ()
                n201 = Decimate 1D Array(w397) -> (w398:dbl[], w399:dbl[], w400:dbl[], w401:dbl[])
                n202 = local write "Soft WARNING level 1: self cleared"(w398) -> ()
                n203 = local write "ERROR level 2 : set IDLING"(w399) -> ()
                n204 = local write "ERROR level 3 : set MOTORING"(w400) -> ()
                n205 = local write "ERROR level 4: STOP and VENT"(w401) -> ()
                n206 = local write "set9056"(FALSE ("set")) -> ()
              }
            }
          }
        }
        "Round Color Box selected" <- w150
        "Selected raster" <- w144
        "Measured value" <- w143
        n207 = Build Array(w46) -> (→"CA50":dbl[][])
        n208 = call <vilib>:"Std Deviation and Variance.vi"("X"=w46) -> ("standard deviation"=→"s":dbl)  [unwired: 1 in, 2 out]
        n209 = call "APC_Warning2DColorMap.vi"("CylPresErrors"=w76, "CylPresWarnings"=w77) -> ("Round Color Box"=w41:u32[][])
        "System error state" <- w41
        "Cylinder pressure state" <- w41
        n210 = Bundle By Name(cluster=T2 {"AI and system state"=[], "Cylinder pressure state"=[], "EMERGENCY STOP"=FALSE} ("Error cluster"), "Cylinder pressure state"=w41, "AI and system state"=w39, "EMERGENCY STOP"="EMERGENCY STOP") -> (w40:T2)
        n211 = case shown="True" "retrieve9056" {
          frame False {
          }
          frame True {
            n212 = local write "Edit mode 9056"(FALSE ("Edit mode 9056")) -> ()
            n213 = shared-variable "NI-cRIO-9049-020A5DED\\APC_SharedVars.lvlib\\9056_RetrieveWarningLimits"(TRUE ("SaveWarningLimitsToINI")) -> ()  [unwired: 1 in, 1 out]
            n214 = local write "retrieve9056"(FALSE ("SaveINI")) -> ()
          }
        }
        n215 = case shown="True" "Clear warnings" {
          frame False {
          }
          frame True {
            n216 = local write "Clear warnings"(FALSE) -> ()
            "Clear warning request" <- TRUE ("Clear warning request")
          }
        }
        n217 = case shown="True" "retrieve9049" {
          frame False {
          }
          frame True {
            w209 = FALSE ("SaveINI")
            n218 = local write "retrieve9049"(w209) -> ()
            n219 = shared-variable "NI-cRIO-9049-020A5DED\\APC_SharedVars.lvlib\\9049_RetrieveWarningLimits"(TRUE ("SaveWarningLimitsToINI")) -> ()  [unwired: 1 in, 1 out]
            n220 = local write "Edit mode 9049"(w209) -> ()
          }
        }
        n221 = shared-variable ".\\APC_PCglobalVars.lvlib\\PC_Global_Errors"(w40) -> ()  [unwired: 1 in, 1 out]
        n222 = shared-variable ".\\APC_PCglobalVars.lvlib\\PC_Global_ListboxVarBroadcastErrors"() -> (w50:u8)  [unwired: 1 in, 1 out]
        n223 = local read "Edit mode 9049"() -> (w36:bool)
        n224 = feedback-in #1("Listbox") -> ()
        n225 = feedback #1() -> (w55:i32)  [unwired: 1 in]
        n226 = And(x="SaveINI9049", y=w36) -> (x .and. y?=w37:bool)
        n227 = Not Equal?(x="Listbox", y=w55) -> (x != y?=w54:bool)
        n228 = case shown="True" w37 {
          frame False {
          }
          frame True {
            w212 = FALSE ("SaveINI")
            n229 = shared-variable "NI-cRIO-9049-020A5DED\\APC_SharedVars.lvlib\\9049_SaveWarningLimitsToINI"(TRUE ("SaveWarningLimitsToINI")) -> ()  [unwired: 1 in, 1 out]
            n230 = local write "Edit mode 9049"(w212) -> ()
            n231 = local write "SaveINI9049"(w212) -> ()
            n232 = local write "retrieve9049"(TRUE ("retrieve9049")) -> ()
          }
        }
        n233 = local read "Edit mode 9056"() -> (w74:bool)
        n234 = case shown="True" w54 {
          frame False {
          }
          frame True {
            n235 = local read "Listbox"() -> (w155:i32)
            n236 = shared-variable "NI-cRIO-9049-020A5DED\\APC_SharedVars.lvlib\\9049_SelectBroadcastVar"(w155) -> ()  [unwired: 1 in, 1 out]
            n237 = shared-variable ".\\APC_PCglobalVars.lvlib\\PC_Global_ListboxVarBroadcastMain"(w155) -> ()  [unwired: 1 in, 1 out]
          }
        }
        n238 = feedback #2() -> (w52:u8)  [unwired: 1 in]
        n239 = feedback-in #2(w50) -> ()
        n240 = And(x="SaveINI9056", y=w74) -> (x .and. y?=w72:bool)
        n241 = Not Equal?(x=w50, y=w52) -> (x != y?=w51:bool)
        n242 = case shown="True" w72 {
          frame False {
            n243 = local write "SaveINI9056"(FALSE ("SaveINI")) -> ()
          }
          frame True {
            n244 = shared-variable "NI-cRIO-9049-020A5DED\\APC_SharedVars.lvlib\\9056_SaveWarningLimitsToINI"(TRUE ("SaveWarningLimitsToINI")) -> ()  [unwired: 1 in, 1 out]
            n245 = local write "SaveINI9056"(FALSE ("SaveINI")) -> ()
            n246 = local write "Edit mode 9056"(FALSE ("Edit mode 9056")) -> ()
            n247 = local write "retrieve9056"(TRUE ("retrieve9056")) -> ()
          }
        }
        n248 = case shown="True" w51 {
          tunnel: w50 -> [_ w153]
          frame False {
          }
          frame True {
            n249 = local write "Listbox"(w153) -> ()
            n250 = property on="Listbox" class="LstBox (strict)"() -> ("Item Names"=w154:string[])  [unwired: 2 in, 2 out]
            n251 = Index Array(array=w154, index=w153) -> (element=w152:string)
            n252 = property on="Waveform Graph" class="WFGraph (strict)"("YScale.NameLbl.Text"=w152) -> ()  [unwired: 2 in, 2 out]
          }
        }
        n253 = local read "Edit mode 9056"() -> (w69:bool)
        n254 = And(x="ReloadINI9056", y=w69) -> (x .and. y?=w70:bool)
        n255 = Wait Until Next ms Multiple(millisecond multiple=u32 200) -> ()  [unwired: 1 out]
        n256 = case shown="True" w70 {
          frame False {
            n257 = local write "ReloadINI9056"(FALSE ("SaveINI")) -> ()
          }
          frame True {
            n258 = shared-variable "NI-cRIO-9049-020A5DED\\APC_SharedVars.lvlib\\9056_LoadWarningsFromINI"(TRUE ("SaveWarningLimitsToINI")) -> ()  [unwired: 1 in, 1 out]
            n259 = local write "ReloadINI9056"(FALSE ("SaveINI")) -> ()
            n260 = local write "Edit mode 9056"(FALSE ("Edit mode 9056")) -> ()
            n261 = local write "retrieve9056"(TRUE ("retrieve9056")) -> ()
          }
        }
        n262 = case shown="True" "Edit mode 9049" {
          frame False {
            w161 = FALSE ("set 2")
            n263 = shared-variable "NI-cRIO-9049-020A5DED\\APC_SharedVars.lvlib\\9049_WarningLevels"() -> (w178:T3)  [unwired: 1 in, 1 out]
            n264 = local write "ReloadINI9049"(w161) -> ()
            n265 = local write "set9049"(w161) -> ()
            n266 = Unbundle By Name(w178) -> ("MaxPCylMaxWarning [bar]"=w177:dbl, "MaxDevFromSelfAvgWarning [bar]"=w176:dbl, "MaxDevFromAvgWarning [bar]"=w175:dbl, "MaxDevFromExpectedIMEPWarning [bar]"=w174:dbl, "MaxIMEPstdWarning [bar]"=w173:dbl, "MAPOmaxWarning [bar/CAD]"=w172:dbl, "CA50maxWarning [CADATDC]"=w171:dbl)
            n267 = Unbundle By Name(w178) -> ("MaxPCylMaxError [bar]"=w170:dbl, "MaxDevFromSelfAvgError [bar]"=w169:dbl, "MaxDevFromAvgError [bar]"=w168:dbl, "MaxDevFromExpectedIMEPError [bar]"=w167:dbl, "MaxIMEPstdError [bar]"=w166:dbl, "MAPOmaxError [bar/CAD]"=w165:dbl, "CA50maxError [CADATDC]"=w164:dbl)
            n268 = Build Array(w177, w176, w175, w174, w173, w172, w171) -> (w163:dbl[])
            n269 = Build Array(w170, w169, w168, w167, w166, w165, w164) -> (w162:dbl[])
            n270 = local write "Warning level : self cleared"(w163) -> ()
            n271 = local write "Error level 2 : set MOTORING"(w162) -> ()
          }
          frame True {
            n272 = case shown="True" "set9049" {
              frame False {
              }
              frame True {
                n273 = local read "Error level 2 : set MOTORING"() -> (w199:dbl[])
                n274 = local read "Warning level : self cleared"() -> (w191:dbl[])
                n275 = local write "set9049"(FALSE ("set 2")) -> ()
                n276 = local write "retrieve9049"(TRUE ("retrieve9049")) -> ()
                n277 = Index Array(array=w191, index #1=0 ("index")) -> (element #1=w192:dbl, element #2=w193:dbl, element #3=w194:dbl, element #4=w195:dbl, element #5=w196:dbl, element #6=w197:dbl, element #7=w198:dbl)  [unwired: 6 in]
                n278 = Index Array(array=w199, index #1=0 ("index")) -> (element #1=w206:dbl, element #2=w205:dbl, element #3=w204:dbl, element #4=w203:dbl, element #5=w202:dbl, element #6=w201:dbl, element #7=w200:dbl)  [unwired: 6 in]
                n279 = Bundle By Name(cluster=T3 {"samples for running IMEP std"=100, "MaxDevFromExpectedIMEPError [bar]"=2.0, "MaxDevFromExpectedIMEPWarning [bar]"=2.0, "MaxDevFromAvgError [bar]"=2.0, "MaxDevFromSelfAvgWarning [bar]"=2.0, "MaxDevFromSelfAvgError [bar]"=2.0, "MaxDevFromAvgWarning [bar]"=2.0, "MaxIMEPstdWarning [bar]"=0.5, "MaxIMEPstdError [bar]"=0.5, "MAPOmaxError [bar/CAD]"=1.0, "MAPOmaxWarning [bar/CAD]"=1.0, "CA50maxError [CADATDC]"=15.0, "CA50maxWarning [CADATDC]"=15.0, "MaxPCylMaxError [bar]"=120.0, "MaxPCylMaxWarning [bar]"=120.0} ("9049_WarningLevels"), "samples for running IMEP std"="cycles for std", "MaxPCylMaxWarning [bar]"=w192, "MaxDevFromSelfAvgWarning [bar]"=w193, "MaxDevFromAvgWarning [bar]"=w194, "MaxDevFromExpectedIMEPWarning [bar]"=w195, "MaxDevFromAvgError [bar]"=w196, "MAPOmaxWarning [bar/CAD]"=w197, "CA50maxWarning [CADATDC]"=w198, "MaxPCylMaxError [bar]"=w206, "MaxDevFromSelfAvgError [bar]"=w205, "MaxDevFromAvgError [bar]"=w204, "MaxDevFromExpectedIMEPError [bar]"=w203, "MaxIMEPstdError [bar]"=w202, "MAPOmaxError [bar/CAD]"=w201, "CA50maxError [CADATDC]"=w200) -> (w190:T3)
                n280 = shared-variable "NI-cRIO-9049-020A5DED\\APC_SharedVars.lvlib\\9049_WarningLevels"(w190) -> (error out=w185:errorcluster)  [unwired: 1 in]
                n281 = shared-variable "NI-cRIO-9049-020A5DED\\APC_SharedVars.lvlib\\9049_SetWarningLimits"(TRUE ("9049SetWarningLimits"), error in=w185) -> ()  [unwired: 1 out]
              }
            }
            n282 = case shown="True" "ReloadINI9049" {
              frame False {
              }
              frame True {
                n283 = local write "retrieve9049"(TRUE ("retrieve9049")) -> ()
                n284 = local write "ReloadINI9049"(FALSE ("ReloadINI")) -> ()
                n285 = shared-variable "NI-cRIO-9049-020A5DED\\APC_SharedVars.lvlib\\9049_LoadWarningsFromINI"(TRUE ("9049LoadWarningsFromINI")) -> ()  [unwired: 1 in, 1 out]
              }
            }
          }
        }
      }
      n286 = while {
        stop <- FALSE stop-if-true
        n287 = local read "Clear warning request"() -> (w31:bool)
        n288 = case shown="True" w31 {
          frame False {
          }
          frame True {
            n289 = local write "Clear warning request"(FALSE ("Clear warning request")) -> ()
            n290 = call "APC_ClearErrorButton.vi"() -> ()  [unwired: 1 in]
          }
        }
        n291 = Wait Until Next ms Multiple(millisecond multiple=u32 200) -> ()  [unwired: 1 out]
      }
    }
    frame #2 {
      n292 = local write "EMERGENCY STOP"(FALSE ("EMERGENCY STOP")) -> ()
    }
  }
